vi "Pulse width to duty cycle.vi"(10 "frequency":dbl, 11 "pulse width (us)":dbl) -> (2 "wait (ms)":dbl, 3 "duty cycle":dbl)   [LabVIEW 2020]
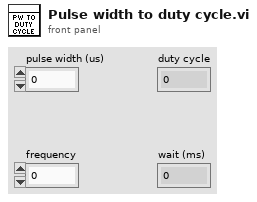
[diagram p1: front panel]
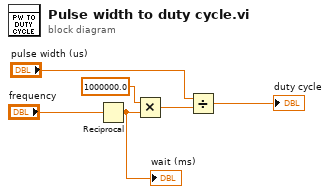
[diagram p0: block diagram]
diagram:
  n1 = Reciprocal(x="frequency") -> (1/x=w4:dbl)
  "wait (ms)" <- w4
  n2 = Multiply(x=1000000.0, y=w4) -> (x*y=w1:dbl)
  n3 = Divide(x="pulse width (us)", y=w1) -> (x/y=→"duty cycle":dbl)
